vi "Switch scanners.vi"() -> ()   [LabVIEW 2016]
doc: "This example switches between 2 different XY scanners.\nIn order to accomplish this, make the following connections if the specified analog outputs are available:\n\n1. Connect scanner 1 to outputs 2 & 3\n2. Connect scanner 2 to outputs 4 & 8\n\nWhen scanner 1 is active, the X/Y scan outputs will be directed to outputs 2 & 3. Outputs 4 & 8 (scanner 2) will be held at it's current position.\n\nThis example doesn't affect the Z scanner, so the user will have to use the necessary functions if he wants to withdraw the tip before switching XY scanners.\n\n- Nanonis Programming Interface -"
uses:
  Nanonis Prog Interface.lvlib
  <userlib>/Nanonis Prog Interface V5/Scan/Piezos/Piezo Calibration Sens Set.vi
panel:
  out "Sens. X (m/V) Active scanner":sgl=6.6667e-10 format="%#_6p"
  out "Sens. Y (m/V) Active scanner":sgl=6.6667e-10 format="%#_6p"
  out "Calib. X (m/V) 2":sgl=6.6667e-10 format="%#_6p"
  out "Calib. Y (m/V) 2":sgl=6.6667e-10 format="%#_6p"
  out "Calib. X (m/V) 1":sgl=6.6667e-10 format="%#_6p"
  out "Calib. Y (m/V) 1":sgl=6.6667e-10 format="%#_6p"
  in  "Gain Y 1":sgl=15.0 caption="Gain Y" min=0 max=1000 format="%#_3f"
  in  "Gain X 1":sgl=15.0 caption="Gain X" min=0 max=1000 format="%#_3f"
  in  "Sens. Y (m/V) 1":sgl=6.6667e-10 caption="Calib. Y (m/V)" format="%#_6p"
  in  "Sens. X (m/V) 1":sgl=6.6667e-10 caption="Calib. X (m/V)" format="%#_6p"
  in  "Scanner name 1":string="Scanner 1" caption="Scanner name"
  in  "Gain Y 2":sgl=15.0 caption="Gain Y" min=0 max=1000 format="%#_3f"
  in  "Gain X 2":sgl=15.0 caption="Gain X" min=0 max=1000 format="%#_3f"
  in  "Sens. Y (m/V) 2":sgl=6.6667e-10 caption="Calib. Y (m/V)" format="%#_6p"
  in  "Sens. X (m/V) 2":sgl=6.6667e-10 caption="Calib. X (m/V)" format="%#_6p"
  in  "Scanner name 2":string="Scanner 2" caption="Scanner name"
  in  "Stop scan":bool
  in  "Start scan":bool
  in  "Initialize outputs":bool
  in  "Switch scanners":bool
  in  "Quit":bool
  in  "Active Scanner":bool=TRUE
  # "1.  Connect scanner 1 to outputs 2 & 3\n2.  Connect scanner 2 to outputs 4 & 8"
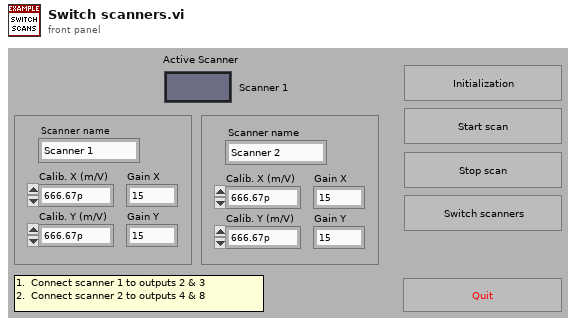
[diagram p1: front panel]
types:
  T1 = enum16{"Initialize outputs", "Settings", "Start scan", "Stop scan", "Switch scanners", "Stop"}
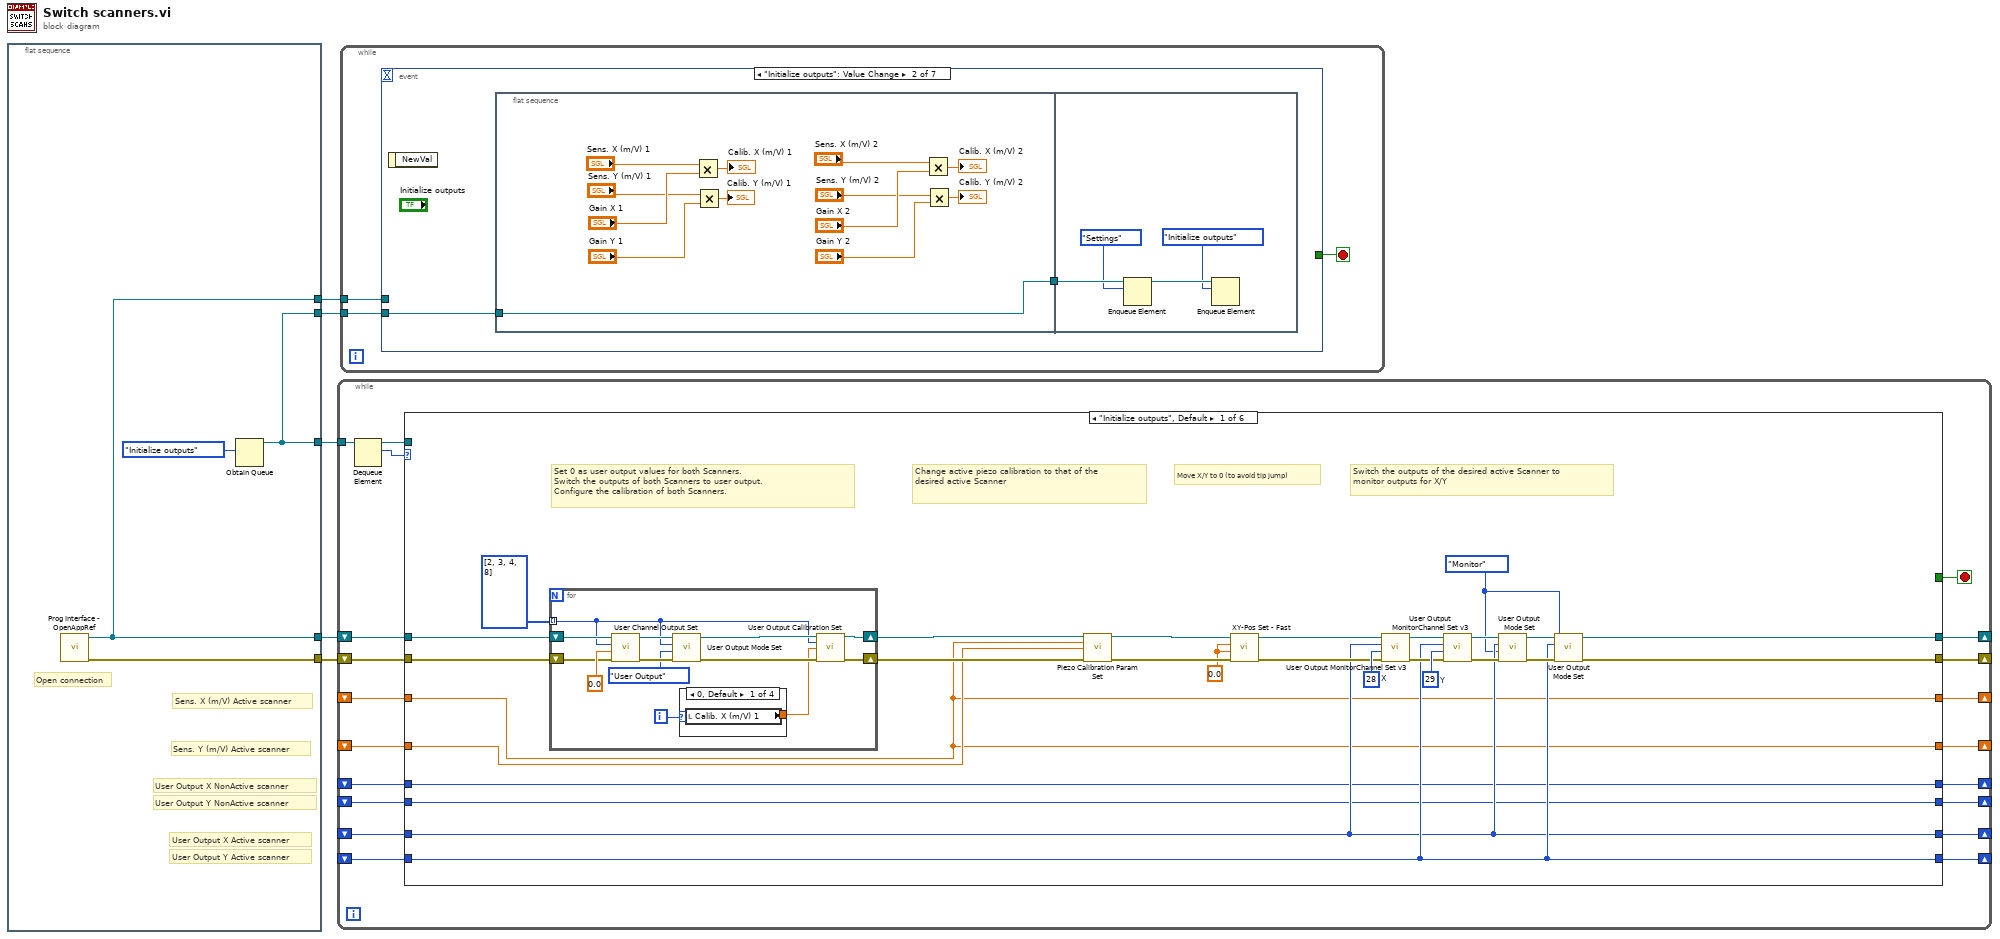
[diagram p0: block diagram]
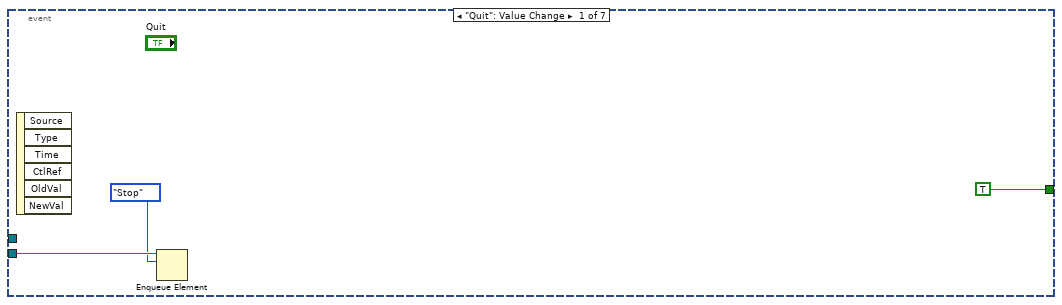
[diagram p2: hidden frame]
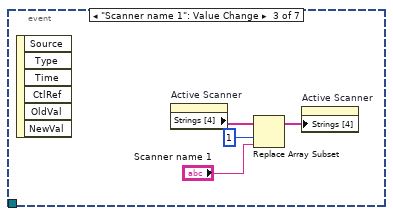
[diagram p3: hidden frame]
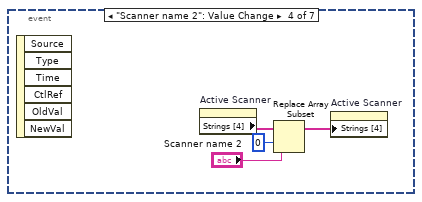
[diagram p4: hidden frame]
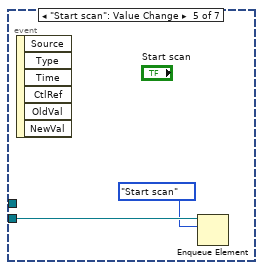
[diagram p5: hidden frame]
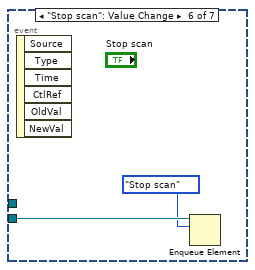
[diagram p6: hidden frame]
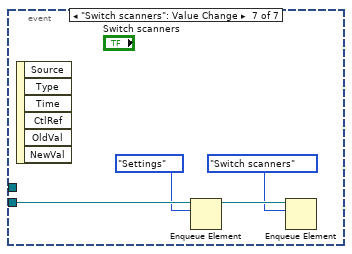
[diagram p7: hidden frame]
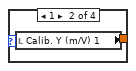
[diagram p8: hidden frame]
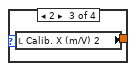
[diagram p9: hidden frame]
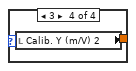
[diagram p10: hidden frame]
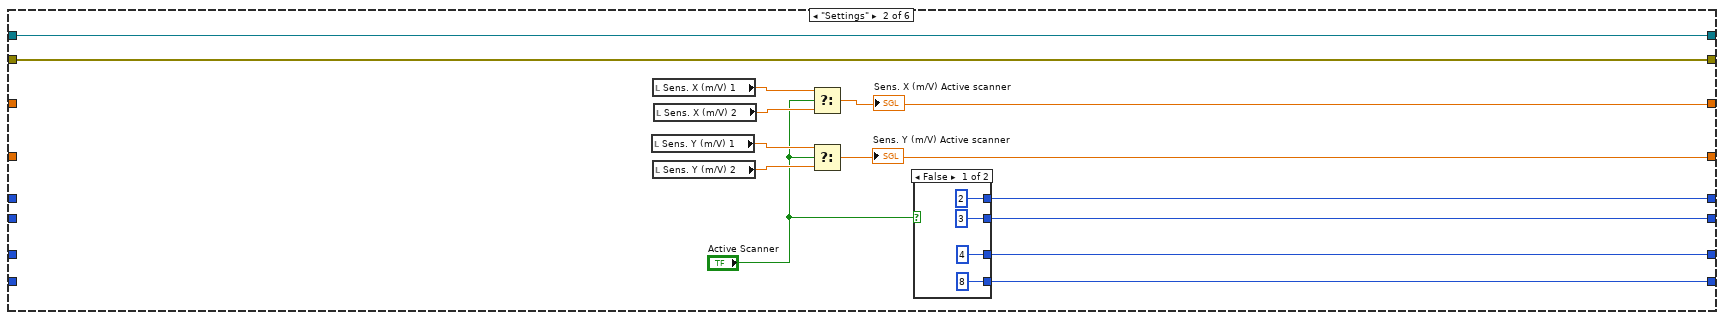
[diagram p11: hidden frame]
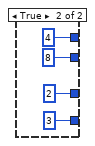
[diagram p12: hidden frame]
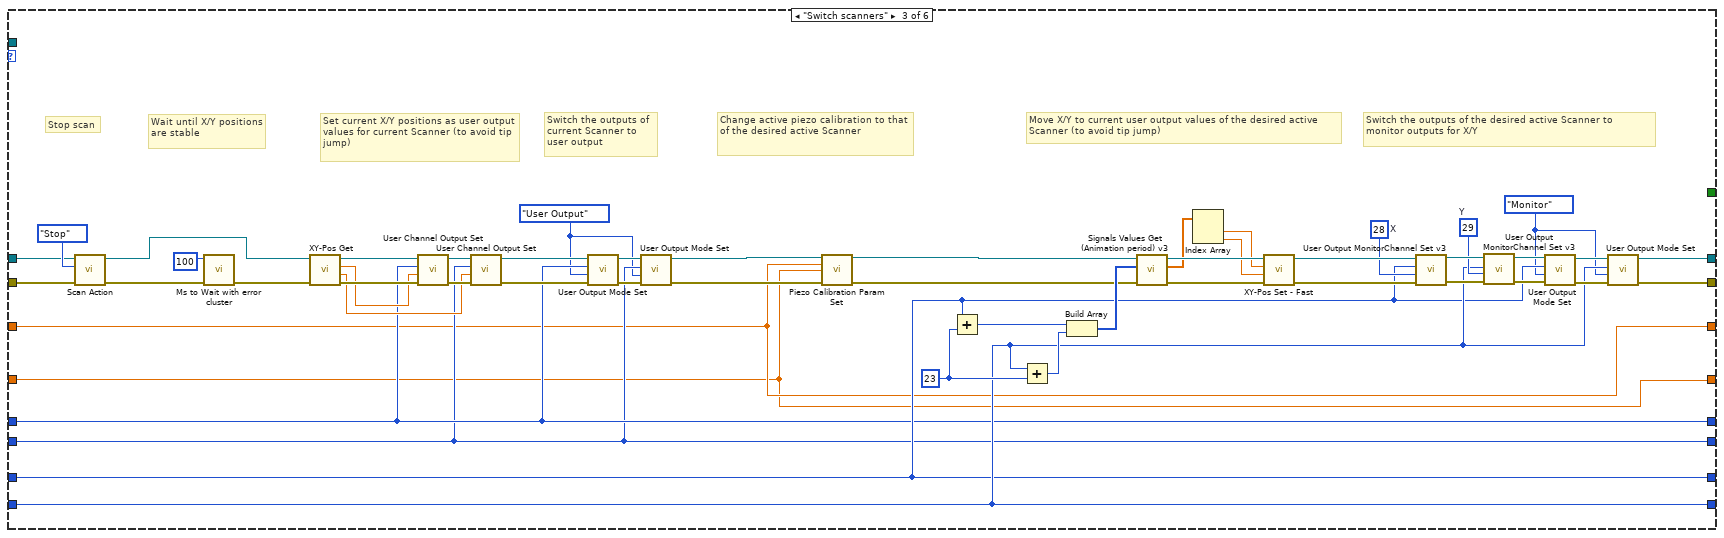
[diagram p13: hidden frame]
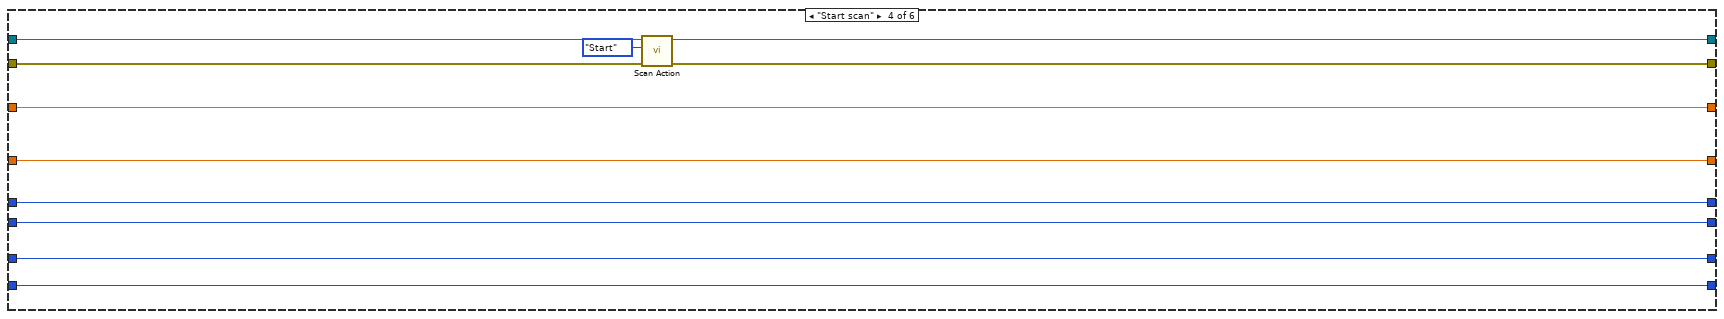
[diagram p14: hidden frame]
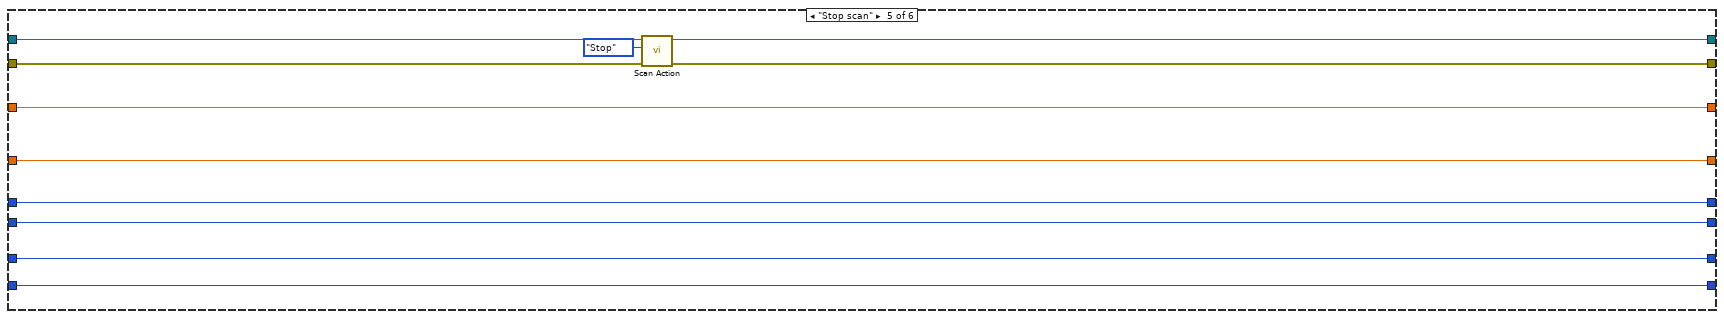
[diagram p15: hidden frame]
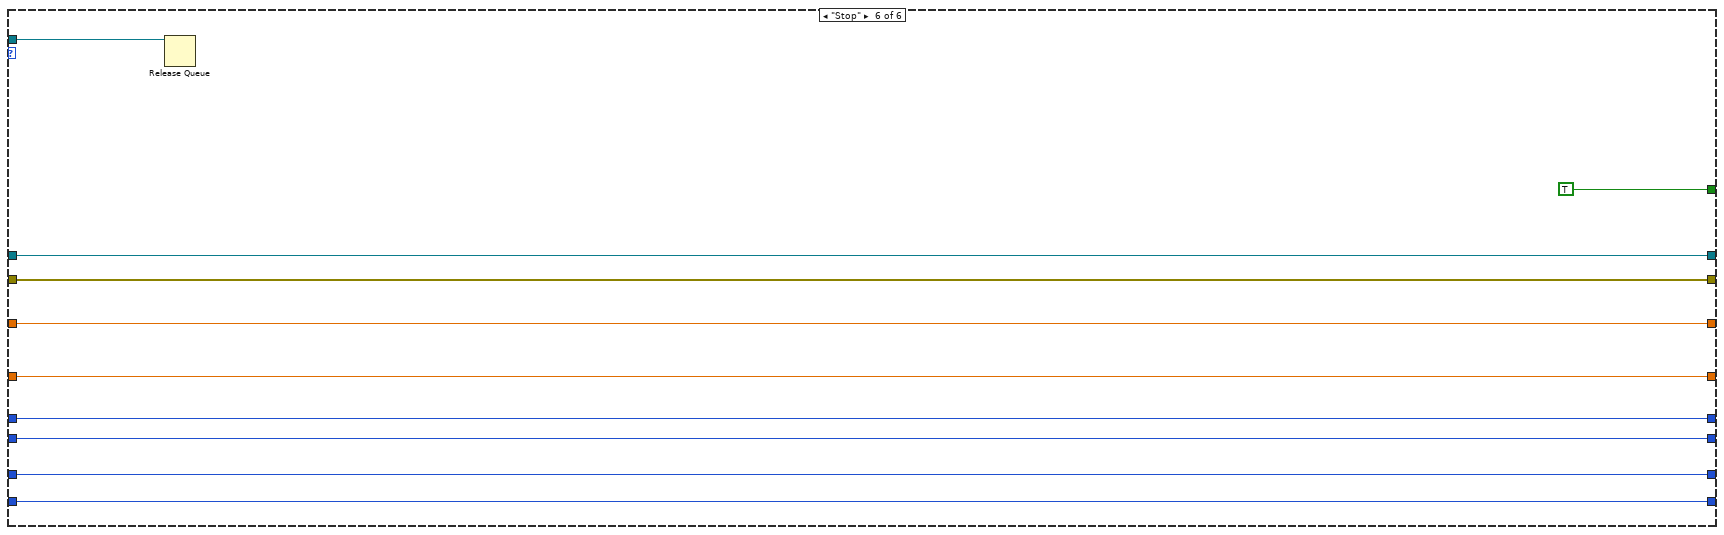
[diagram p16: hidden frame]
diagram:
  n1 = flat-sequence {
    tunnel: [w8] -> w5
    tunnel: [w9] -> w4
    tunnel: [w8] -> w3
    tunnel: [w6] -> w2
    tunnel: [w6] -> w1
    frame #0 {
      # "User Output Y NonActive scanner"
      # "User Output X NonActive scanner"
      # "User Output Y Active scanner"
      # "User Output X Active scanner"
      # "Sens. Y (m/V) Active scanner"
      # "Sens. X (m/V) Active scanner"
      # "Open connection"
      n2 = call <userlib>:"Prog Interface - OpenAppRef.vi"() -> ("Error out"=w9:errorcluster, "Application reference"=w8:refnum<vi>)  [unwired: 6 in]
      n3 = Obtain Queue(element data type=T1."Initialize outputs" ("states")) -> (queue out=w6:refnum<queue>)  [unwired: 4 in, 2 out]
    }
  }
  n4 = while {
    shift-right: [w26] -> _
    shift-left: w5 -> [w29]
    shift-right: [w27] -> _
    shift-left: w4 -> [w28]
    tunnel: w2 -> [w25]
    shift-right: [w21] -> _
    shift-left: _ -> [w11]
    shift-right: [w20] -> _
    shift-left: _ -> [w10]
    shift-right: [w19] -> _
    shift-left: _ -> [w12]
    shift-right: [w18] -> _
    shift-left: _ -> [w13]
    shift-right: [w17] -> _
    shift-left: _ -> [w14]
    shift-right: [w16] -> _
    shift-left: _ -> [w15]
    stop <- w22 stop-if-true
    n5 = Dequeue Element(queue=w25) -> (queue out=w23:refnum<queue>, element=w24:T1)  [unwired: 2 in, 2 out]
    n6 = case shown="\"Initialize outputs\", Default" w24 {
      tunnel: w29 -> [w40 w76 w110 w154 w165 w174]
      tunnel: w28 -> [w39 w75 w109 w153 w164 w173]
      tunnel: [w37 w75 w108 w151 w162 w173] -> w27
      tunnel: [w38 w76 w107 w152 w163 w174] -> w26
      tunnel: w23 -> [_ _ _ _ _ w176]
      tunnel: [_ _ _ _ _ TRUE] -> w22
      tunnel: [w34 w82 w101 w146 w157 w168] -> w21
      tunnel: [w35 w81 w102 w145 w156 w167] -> w20
      tunnel: [w31 w80 w99 w147 w158 w169] -> w19
      tunnel: [w32 w79 w100 w148 w159 w170] -> w18
      tunnel: [w33 w78 w97 w149 w160 w171] -> w17
      tunnel: [w33 w77 w98 w150 w161 w172] -> w16
      tunnel: w15 -> [w33 _ w98 w150 w161 w172]
      tunnel: w14 -> [w36 _ w97 w149 w160 w171]
      tunnel: w13 -> [w32 _ w100 w148 w159 w170]
      tunnel: w12 -> [w31 _ w99 w147 w158 w169]
      tunnel: w11 -> [w34 _ w101 w146 w157 w168]
      tunnel: w10 -> [w35 _ w102 w145 w156 w167]
      frame "Initialize outputs", Default {
        w30 = enum8{"User Output", "Monitor", "Calc. Signal"}."Monitor" ("Output Mode (UserOut)")
        w56 = i8 29  # Y
        w55 = i8 28  # X
        w42 = sgl 0.0 ("X (m)")
        # "Set 0 as user output values for both Scanners.\nSwitch the outputs of both Scanners to user output.\nConfigure the calibration of both Scanners."
        # "Change active piezo calibration to that of the desired active Scanner"
        # "Move X/Y to 0 (to avoid tip jump)"
        # "Switch the outputs of the desired active Scanner to monitor outputs for X/Y"
        n7 = for {
          shift-right: [w62] -> w44
          shift-left: w39 -> [w67]
          shift-right: [w63] -> w43
          shift-left: w40 -> [w65]
          tunnel: u8[] [2, 3, 4, 8] -> [w58] mode=indexing
          i -> [w60]
          n8 = call <userlib>:"User Channel Output Set.vi"("error in (no error)"=w67, "Output value (physical unit)"=sgl 0.0, "User output channel"=w58, "Application ref in"=w65) -> ("error out"=w68:errorcluster, "Application ref out"=w66:refnum<vi>)  [unwired: 5 in]
          n9 = call <userlib>:"User Output Mode Set.vi"("error in (no error)"=w68, "Output Mode (UserOut)"=enum8{"User Output", "Monitor", "Calc. Signal"}."User Output", "User output channel"=w58, "Application ref in"=w66) -> ("error out"=w61:errorcluster, "Application ref out"=w64:refnum<vi>)  [unwired: 5 in]
          n10 = case shown="0, Default" w60 {
            tunnel: [w70 w71 w72 w73] -> w59
            frame 0, Default {
              n11 = local read "Calib. X (m/V) 1"() -> (w70:sgl)
            }
            frame 1 {
              n12 = local read "Calib. Y (m/V) 1"() -> (w71:sgl)
            }
            frame 2 {
              n13 = local read "Calib. X (m/V) 2"() -> (w72:sgl)
            }
            frame 3 {
              n14 = local read "Calib. Y (m/V) 2"() -> (w73:sgl)
            }
          }
          n15 = call <userlib>:"User Output Calibration Set.vi"("Application ref in"=w64, "User output channel"=w58, "Calibration (per Volt)"=w59, "error in (no error)"=w61) -> ("Application ref out"=w63:refnum<vi>, "error out"=w62:errorcluster)  [unwired: 10 in]
        }
        n16 = call-poly "Piezo Calibration Param Set.vi"("Application ref in"=w43, "Calib. X (m/V) (NaN=no change)"=w33, "Calib. Y (m/V) (NaN=no change)"=w36, "error in (no error)"=w44) -> ("Application ref out"=w46:refnum<vi>, "error out"=w45:errorcluster)  [unwired: 10 in]
        n17 = call <userlib>:"XY-Pos Set - Fast.vi"("error in (no error)"=w45, "Y (m)"=w42, "X (m)"=w42, "Application ref in"=w46) -> ("error out"=w51:errorcluster, "Application ref out"=w50:refnum<vi>)  [unwired: 5 in]
        n18 = call <userlib>:"User Output MonitorChannel Set v3.vi"("error in (no error)"=w51, "Monitor channel index (0-127)"=w55, "User output channel"=w34, "Application ref in"=w50) -> ("error out"=w48:errorcluster, "Application ref out"=w52:refnum<vi>)  [unwired: 5 in]
        n19 = call <userlib>:"User Output MonitorChannel Set v3.vi"("error in (no error)"=w48, "Monitor channel index (0-127)"=w56, "User output channel"=w35, "Application ref in"=w52) -> ("error out"=w47:errorcluster, "Application ref out"=w53:refnum<vi>)  [unwired: 5 in]
        n20 = call <userlib>:"User Output Mode Set.vi"("error in (no error)"=w47, "Output Mode (UserOut)"=w30, "User output channel"=w34, "Application ref in"=w53) -> ("error out"=w49:errorcluster, "Application ref out"=w54:refnum<vi>)  [unwired: 5 in]
        n21 = call <userlib>:"User Output Mode Set.vi"("error in (no error)"=w49, "Output Mode (UserOut)"=w30, "User output channel"=w35, "Application ref in"=w54) -> ("error out"=w37:errorcluster, "Application ref out"=w38:refnum<vi>)  [unwired: 5 in]
      }
      frame "Settings" {
        n22 = local read "Sens. Y (m/V) 1"() -> (w85:sgl)
        n23 = local read "Sens. X (m/V) 1"() -> (w86:sgl)
        n24 = local read "Sens. Y (m/V) 2"() -> (w83:sgl)
        n25 = local read "Sens. X (m/V) 2"() -> (w84:sgl)
        n26 = Select(t=w86, s="Active Scanner", f=w84) -> (s? t:f=w77:sgl)
        "Sens. X (m/V) Active scanner" <- w77
        n27 = Select(t=w85, s="Active Scanner", f=w83) -> (s? t:f=w78:sgl)
        "Sens. Y (m/V) Active scanner" <- w78
        n28 = case shown="False" "Active Scanner" {
          tunnel: [u8 8 ("Output channel Y (1-8)") u8 3 ("Output channel Y (1-8)")] -> w81
          tunnel: [u8 4 ("Output channel Y (1-8)") u8 2 ("Output channel Y (1-8)")] -> w82
          tunnel: [u8 2 ("Output channel Y (1-8)") u8 4 ("Output channel Y (1-8)")] -> w79
          tunnel: [u8 3 ("Output channel Y (1-8)") u8 8 ("Output channel Y (1-8)")] -> w80
          frame False {
          }
          frame True {
          }
        }
      }
      frame "Switch scanners" {
        w95 = enum8{"User Output", "Monitor", "Calc. Signal"}."User Output" ("Output Mode (UserOut)")
        w96 = enum8{"User Output", "Monitor", "Calc. Signal"}."Monitor" ("Output Mode (UserOut)")
        w103 = u8 23 ("y")
        w104 = i8 29  # Y
        w120 = i8 28  # X
        # "Switch the outputs of the desired active Scanner to monitor outputs for X/Y"
        # "Move X/Y to current user output values of the desired active Scanner (to avoid tip jump)"
        # "Change active piezo calibration to that of the desired active Scanner"
        # "Set current X/Y positions as user output values for current Scanner (to avoid tip jump)"
        # "Switch the outputs of current Scanner to user output"
        # "Wait until X/Y positions \nare stable"
        # "Stop scan"
        n29 = call <userlib>:"Scan Action.vi"("error in (no error)"=w109, "Scan action (Start)"=enum16{"Start", "Stop", "Pause", "Resume"}."Stop", "Application ref in"=w110) -> ("error out"=w143:errorcluster, "Application ref out"=w142:refnum<vi>)  [unwired: 6 in]
        n30 = call "Ms to Wait with error cluster.vi"("error in (no error)"=w143, "milliseconds to wait"=u32 100 ("ms to wait after stop scan")) -> ("error out"=w141:errorcluster)  [unwired: 4 in, 1 out]
        n31 = call <userlib>:"XY-Pos Get.vi"("error in (no error)"=w141, "Application ref in"=w142) -> ("error out"=w140:errorcluster, "Y (m)"=w135:sgl, "X (m)"=w136:sgl, "Application ref out"=w139:refnum<vi>)  [unwired: 5 in]
        n32 = call <userlib>:"User Channel Output Set.vi"("error in (no error)"=w140, "Output value (physical unit)"=w136, "User output channel"=w100, "Application ref in"=w139) -> ("error out"=w138:errorcluster, "Application ref out"=w137:refnum<vi>)  [unwired: 5 in]
        n33 = call <userlib>:"User Channel Output Set.vi"("error in (no error)"=w138, "Output value (physical unit)"=w135, "User output channel"=w99, "Application ref in"=w137) -> ("error out"=w133:errorcluster, "Application ref out"=w134:refnum<vi>)  [unwired: 5 in]
        n34 = call <userlib>:"User Output Mode Set.vi"("error in (no error)"=w133, "Output Mode (UserOut)"=w95, "User output channel"=w100, "Application ref in"=w134) -> ("error out"=w132:errorcluster, "Application ref out"=w131:refnum<vi>)  [unwired: 5 in]
        n35 = call <userlib>:"User Output Mode Set.vi"("error in (no error)"=w132, "Output Mode (UserOut)"=w95, "User output channel"=w99, "Application ref in"=w131) -> ("error out"=w129:errorcluster, "Application ref out"=w130:refnum<vi>)  [unwired: 5 in]
        n36 = call-poly "Piezo Calibration Param Set.vi"("Application ref in"=w130, "Calib. X (m/V) (NaN=no change)"=w98, "Calib. Y (m/V) (NaN=no change)"=w97, "error in (no error)"=w129) -> ("Application ref out"=w106:refnum<vi>, "error out"=w105:errorcluster)  [unwired: 10 in]
        n37 = Add(x=w101, y=w103) -> (x+y=w117:u8)
        n38 = Add(x=w102, y=w103) -> (x+y=w116:u8)
        n39 = Build Array(w117, w116) -> (w115:u8[])
        n40 = call <userlib>:"Signals Values Get (Animation period) v3.vi"("error in (no error)"=w105, "Signals indexes (0-127)"=w115, "Application ref in"=w106) -> ("error out"=w119:errorcluster, "Signals Values"=w114:sgl[], "Application ref out"=w118:refnum<vi>)  [unwired: 5 in]
        n41 = Index Array(array=w114) -> (element #1=w113:sgl, element #2=w112:sgl)  [unwired: 2 in]
        n42 = call <userlib>:"XY-Pos Set - Fast.vi"("error in (no error)"=w119, "Y (m)"=w112, "X (m)"=w113, "Application ref in"=w118) -> ("error out"=w125:errorcluster, "Application ref out"=w126:refnum<vi>)  [unwired: 5 in]
        n43 = call <userlib>:"User Output MonitorChannel Set v3.vi"("error in (no error)"=w125, "Monitor channel index (0-127)"=w120, "User output channel"=w101, "Application ref in"=w126) -> ("error out"=w124:errorcluster, "Application ref out"=w123:refnum<vi>)  [unwired: 5 in]
        n44 = call <userlib>:"User Output MonitorChannel Set v3.vi"("error in (no error)"=w124, "Monitor channel index (0-127)"=w104, "User output channel"=w102, "Application ref in"=w123) -> ("error out"=w121:errorcluster, "Application ref out"=w122:refnum<vi>)  [unwired: 5 in]
        n45 = call <userlib>:"User Output Mode Set.vi"("error in (no error)"=w121, "Output Mode (UserOut)"=w96, "User output channel"=w101, "Application ref in"=w122) -> ("error out"=w128:errorcluster, "Application ref out"=w127:refnum<vi>)  [unwired: 5 in]
        n46 = call <userlib>:"User Output Mode Set.vi"("error in (no error)"=w128, "Output Mode (UserOut)"=w96, "User output channel"=w102, "Application ref in"=w127) -> ("error out"=w108:errorcluster, "Application ref out"=w107:refnum<vi>)  [unwired: 5 in]
      }
      frame "Start scan" {
        n47 = call <userlib>:"Scan Action.vi"("error in (no error)"=w153, "Scan action (Start)"=enum16{"Start", "Stop", "Pause", "Resume"}."Start", "Application ref in"=w154) -> ("error out"=w151:errorcluster, "Application ref out"=w152:refnum<vi>)  [unwired: 6 in]
      }
      frame "Stop scan" {
        n48 = call <userlib>:"Scan Action.vi"("error in (no error)"=w164, "Scan action (Start)"=enum16{"Start", "Stop", "Pause", "Resume"}."Stop", "Application ref in"=w165) -> ("error out"=w162:errorcluster, "Application ref out"=w163:refnum<vi>)  [unwired: 6 in]
      }
      frame "Stop" {
        n49 = Release Queue(queue=w176) -> ()  [unwired: 2 in, 3 out]
      }
    }
  }
  n50 = while {
    tunnel: w3 -> [w179]
    tunnel: w1 -> [w177]
    stop <- w178 stop-if-true
    n51 = event shown="[1] \"Initialize outputs\": Value Change" {
      selector: _ -> [_ _ _ _ _ _ _]
      dyn-events: _ -> [_ _ _ _ _ _ _]
      timeout: _ -> [_ _ _ _ _ _ _]
      tunnel: w179 -> [_ _ _ _ _ _ _]
      tunnel: [TRUE _ _ _ _ _ _] -> w178
      tunnel: w177 -> [w182 w183 _ _ w211 w213 w217]
      event "Quit": Value Change {
        n52 = event-data() -> ()  [unwired: 1 in, 6 out]
        n53 = Enqueue Element(queue=w182, element=T1."Stop") -> ()  [unwired: 2 in, 3 out]
      }
      event "Initialize outputs": Value Change {
        n54 = event-data() -> ()  [unwired: 1 in, 1 out]
        n55 = flat-sequence {
          tunnel: [w189] -> w184
          tunnel: w183 -> [w189]
          tunnel: w184 -> [w201]
          frame #0 {
            n56 = Multiply(x="Sens. X (m/V) 1", y="Gain X 1") -> (x*y=→"Calib. X (m/V) 1":sgl)
            n57 = Multiply(x="Sens. Y (m/V) 1", y="Gain Y 1") -> (x*y=→"Calib. Y (m/V) 1":sgl)
            n58 = Multiply(x="Sens. X (m/V) 2", y="Gain X 2") -> (x*y=→"Calib. X (m/V) 2":sgl)
            n59 = Multiply(x="Sens. Y (m/V) 2", y="Gain Y 2") -> (x*y=→"Calib. Y (m/V) 2":sgl)
          }
          frame #1 {
            n60 = Enqueue Element(queue=w201, element=T1."Settings") -> (queue out=w199:refnum<queue>)  [unwired: 2 in, 2 out]
            n61 = Enqueue Element(queue=w199, element=T1."Initialize outputs") -> ()  [unwired: 2 in, 3 out]
          }
        }
      }
      event "Scanner name 1": Value Change {
        n62 = event-data() -> ()  [unwired: 1 in, 6 out]
        n63 = property on="Active Scanner" class="Bool (strict)"() -> ("Strings [4]"=w205:string[])  [unwired: 2 in, 2 out]
        n64 = Replace Array Subset(array=w205, new element="Scanner name 1", index=1) -> (w204:string[])
        n65 = property on="Active Scanner" class="Bool (strict)"("Strings [4]"=w204) -> ()  [unwired: 2 in, 2 out]
      }
      event "Scanner name 2": Value Change {
        n66 = event-data() -> ()  [unwired: 1 in, 6 out]
        n67 = property on="Active Scanner" class="Bool (strict)"() -> ("Strings [4]"=w209:string[])  [unwired: 2 in, 2 out]
        n68 = Replace Array Subset(array=w209, new element="Scanner name 2", index=0) -> (w208:string[])
        n69 = property on="Active Scanner" class="Bool (strict)"("Strings [4]"=w208) -> ()  [unwired: 2 in, 2 out]
      }
      event "Start scan": Value Change {
        n70 = event-data() -> ()  [unwired: 1 in, 6 out]
        n71 = Enqueue Element(queue=w211, element=T1."Start scan") -> ()  [unwired: 2 in, 3 out]
      }
      event "Stop scan": Value Change {
        n72 = event-data() -> ()  [unwired: 1 in, 6 out]
        n73 = Enqueue Element(queue=w213, element=T1."Stop scan") -> ()  [unwired: 2 in, 3 out]
      }
      event "Switch scanners": Value Change {
        n74 = event-data() -> ()  [unwired: 1 in, 6 out]
        n75 = Enqueue Element(queue=w217, element=T1."Settings") -> (queue out=w215:refnum<queue>)  [unwired: 2 in, 2 out]
        n76 = Enqueue Element(queue=w215, element=T1."Switch scanners") -> ()  [unwired: 2 in, 3 out]
      }
    }
  }
